vi "Parse RS232 Data to String.vi"(9 "AML end byte":i32, 10 "AML start byte":i32, 11 "bytes in":string) -> (2 "string data":string, 3 "bytes out":string)   [LabVIEW 2019, in "PGC2D.lvlib"]
uses:
  PGC2D.lvlib
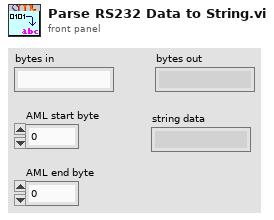
[diagram p1: front panel]
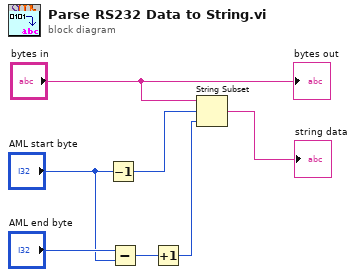
[diagram p0: block diagram]
diagram:
  n1 = Decrement(x="AML start byte") -> (x-1=w1:i32)
  n2 = Subtract(x="AML end byte", y="AML start byte") -> (x-y=w4:i32)
  n3 = Increment(x=w4) -> (x+1=w2:i32)
  n4 = String Subset(string="bytes in", offset (0)=w1, length (rest)=w2) -> (substring=→"string data":string)
  "bytes out" <- "bytes in"
